vi "ACT_Loop.vi"() -> ()   [LabVIEW 2023, in "RingPlacer_ACT.lvlib"]
uses:
  RingPlacer_ACT.lvlib
  Cluster_CMD_ACT_Data.ctl
  ENUM_Shooter_Mode.ctl
  Cluster_Shooter Status.ctl
  Shooter/Cluster_Speed Sensor Values.ctl
  Shooter/Cluster_Velocity Values.ctl
  Shooter/Cluster_Voltage Values.ctl
  ENUM_ACT_State.ctl
  <vilib>/Rock Robotics/WPI/MotorControl/WPI_MotorControlDeviceRef.ctl
  <vilib>/Rock Robotics/WPI/MotorControl/WPI_MotorControlType.ctl
  <vilib>/Rock Robotics/SystemInterfaces/DIO/FPGA_DIOPWMChannel.ctl
  <vilib>/Rock Robotics/WPI/PWM/WPI_PWMDeadband.ctl
  <vilib>/Rock Robotics/SystemInterfaces/DIO/FPGA_DIOChannel.ctl
  <vilib>/Rock Robotics/WPI/ThirdParty/REV Robotics/REVLib/Typedef/Spark MAX Control Type.ctl
  ENUM_ACT_Action.ctl
  <vilib>/Rock Robotics/WPI/ThirdParty/REV Robotics/REVLib/Typedef/Spark MAX Idle Mode.ctl
  RoboRIO Utilities/Global_STOP.vi
  Global_CMD_ACT_Data In.vi
  Global_ACT_Data Out.vi
  Shooter/Shooter_ACT.lvlib
panel:
  out "Motor Status":T1
  out "Target RPM":dbl
  out "Input DBL Data":T5
  out "Output DBL Data":dbl
  out "Cycle Time (S)":dbl format="%.3g"
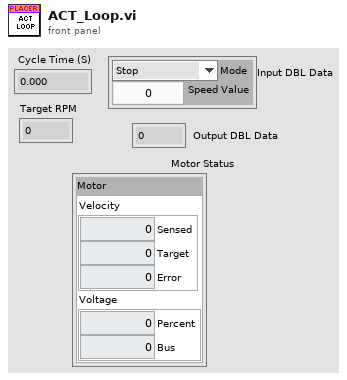
[diagram p1: front panel]
types:
  T1 = typedef "RingPlacer_ACT.lvlib/Cluster_Shooter Status.ctl" = cluster{"Motor":T2}
  T2 = typedef "Cluster_Speed Sensor Values.ctl" = cluster{"Velocity":T3, "Voltage":T4}
  T3 = typedef "Shooter_ACT.lvlib/Cluster_Velocity Values.ctl" = cluster{"Sensed":dbl, "Target":dbl, "Error":dbl}
  T4 = typedef "Shooter_ACT.lvlib/Cluster_Voltage Values.ctl" = cluster{"Percent":dbl, "Bus":dbl}
  T5 = typedef "RingPlacer_ACT.lvlib/Cluster_CMD_ACT_Data.ctl" = cluster{"Mode":T6, "Speed Value":dbl}
  T6 = typedef "RingPlacer_ACT.lvlib/ENUM_Shooter_Mode.ctl" = enum16{"Stop", "Speed Percent", "Speed RPM"}
  T7 = typedef "Spark MAX Control Type.ctl" = enum16{"Percent VBus", "Voltage", "Velocity", "Position", "Smart Motion", "Current", "Smart Velocity"}
  T8 = typedef "WPI_MotorControlDeviceRef.ctl" = cluster{"DeviceStatus":errorcluster, "Type":T9, "PWM":cluster{"PWM Channel":T10, "DeadBand":T11}, "CAN":cluster{"Device Number":u8, "SetOutput VI Ref":variant, "GetOutput VI Ref":variant, "Enable VI Ref":variant, "Disable VI Ref":variant, "Data":variant}, "Invert":bool, "DIO PWM":cluster{"PWM \"Enable\" Channel":T10, "DIOChannel":T12, "PWM Rate":dbl}}
  T9 = typedef "WPI_MotorControlType.ctl" = enum16{"PWM", "CAN", "DIO PWM"}
  T10 = typedef "FPGA_DIOPWMChannel.ctl" = enum8{"PWM 0", "PWM 1", "PWM 2", "PWM 3", "PWM 4", "PWM 5", "PWM 6", "PWM 7", "PWM 8", "PWM 9", "PWM MXP 0", "PWM MXP 1", "PWM MXP 2", "PWM MXP 3", "PWM MXP 4", "PWM MXP 5", "PWM MXP 6", "PWM MXP 7", "PWM MXP 8", "PWM MXP 9", "Invalid"}
  T11 = typedef "WPI_PWMDeadband.ctl" = cluster{"Name":string, "maxPositivePwm":i32, "minPositivePwm":i32, "centerPwm":i32, "maxNegativePwm":i32, "minNegativePwm":i32, "angularRange":u16}
  T12 = typedef "FPGA_DIOChannel.ctl" = enum8{"DIO 0", "DIO 1", "DIO 2", "DIO 3", "DIO 4", "DIO 5", "DIO 6", "DIO 7", "DIO 8", "DIO 9", "DIO MXP 0", "DIO MXP 1", "DIO MXP 2", "DIO MXP 3", "DIO MXP 4", "DIO MXP 5", "DIO MXP 6", "DIO MXP 7", "DIO MXP 8", "DIO MXP 9", "DIO MXP 10", "DIO MXP 11", "DIO MXP 12", "DIO MXP 13", "DIO MXP 14", "DIO MXP 15", "SPI Port CS1", "SPI Port CS2", "SPI Port CS3", "SPI Port MISO", "SPI Port MOSI", "Invalid"}
  T13 = typedef "RingPlacer_ACT.lvlib/ENUM_ACT_State.ctl" = enum16{"Starting", "Stopping", "Shooting", "Shutdown"}
  T14 = typedef "RingPlacer_ACT.lvlib/ENUM_ACT_Action.ctl" = enum16{"No Action", "Reset Time", "Reset All", "Setup Motors", "Setup Sensors", "Stop", "Set Speed RPM", "Set Speed Percent"}
  T15 = cluster{"Motor Ref":T8, "State":T13, "Previous State":T13, "Current Time":timestamp, "Previous Time":timestamp, "Start Time":timestamp, "Target Time (ms)":u32, "Cycle Time(S)":dbl, "ACT Input":T5, "Motor Value":dbl, "Control Mode":T7, "Target RPM":dbl, "Motor Status":T1}
  T16 = typedef "Spark MAX Idle Mode.ctl" = enum16{"Coast", "Brake"}
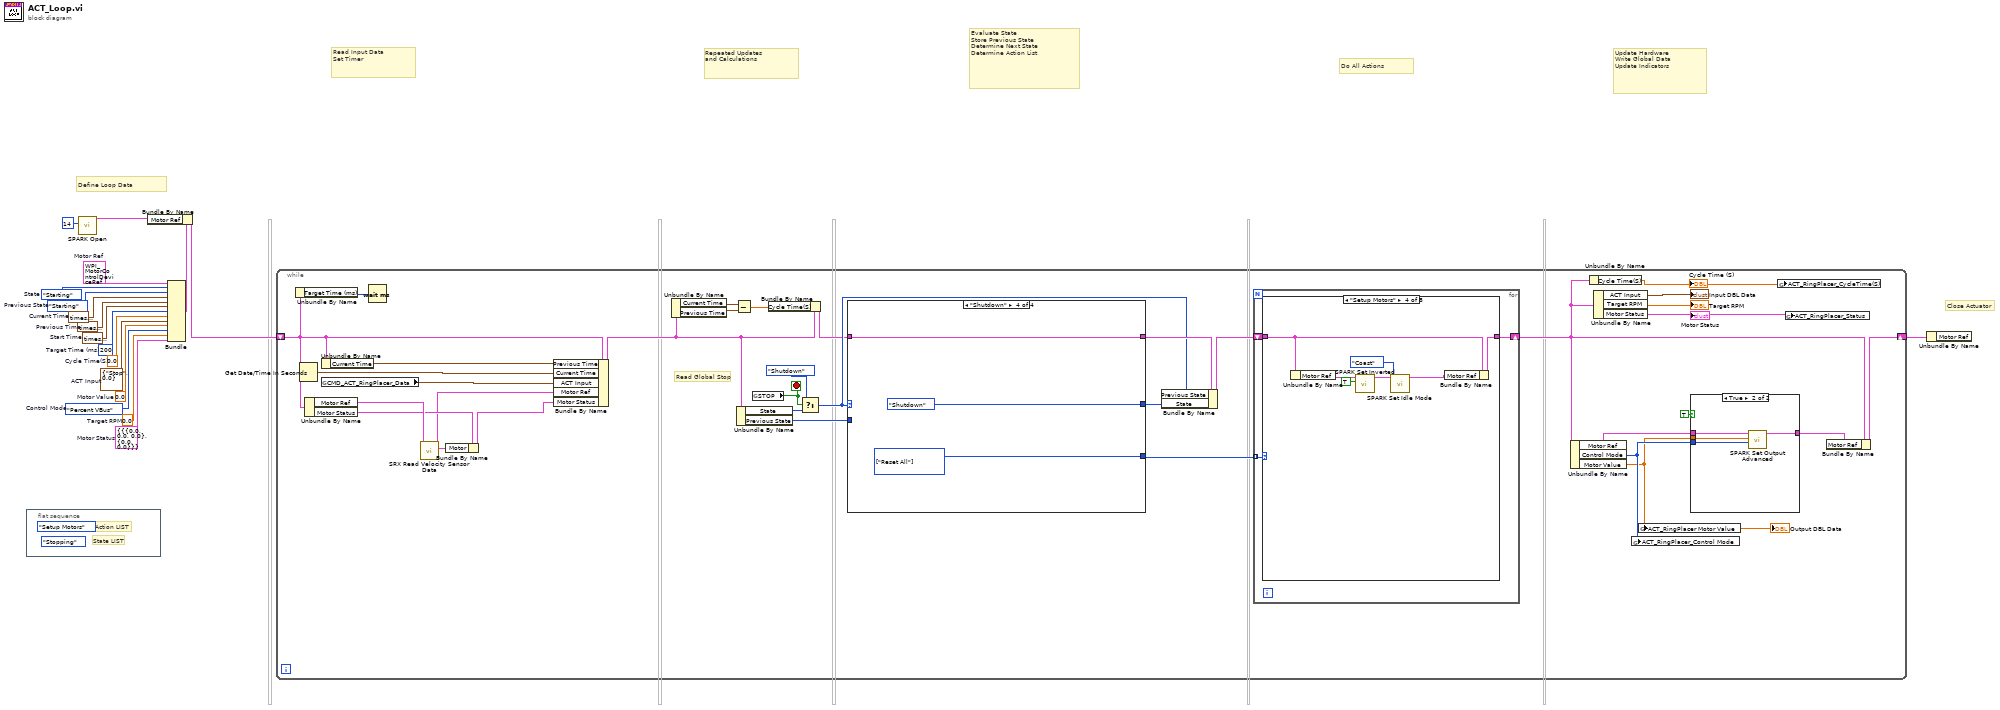
[diagram p0: block diagram]
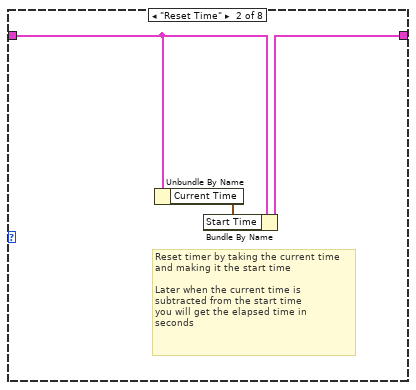
[diagram p4: hidden frame]
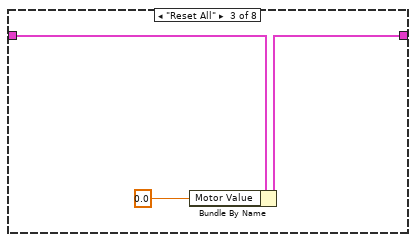
[diagram p5: hidden frame]
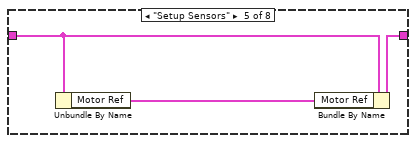
[diagram p6: hidden frame]
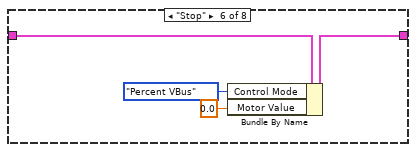
[diagram p7: hidden frame]
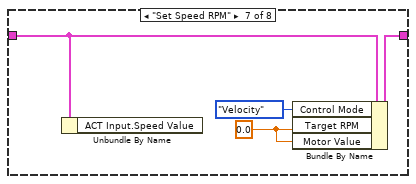
[diagram p8: hidden frame]
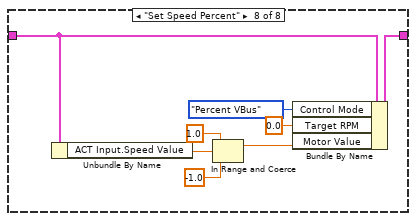
[diagram p9: hidden frame]
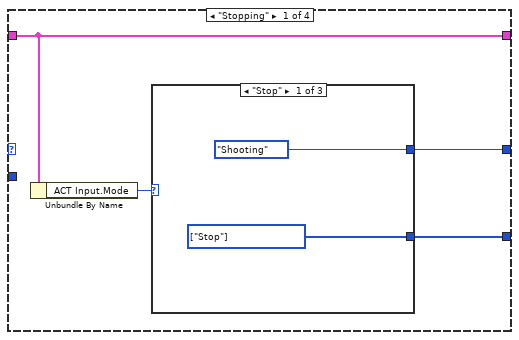
[diagram p10: hidden frame]
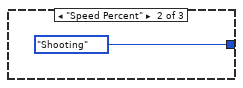
[diagram p11: hidden frame]
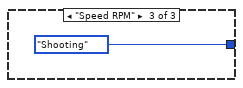
[diagram p12: hidden frame]
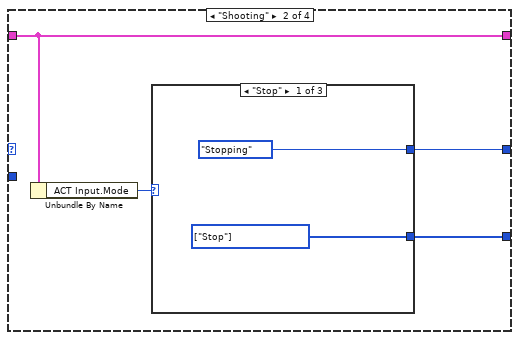
[diagram p13: hidden frame]
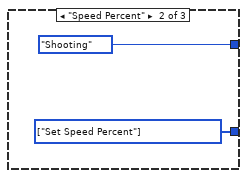
[diagram p14: hidden frame]
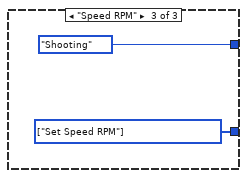
[diagram p15: hidden frame]
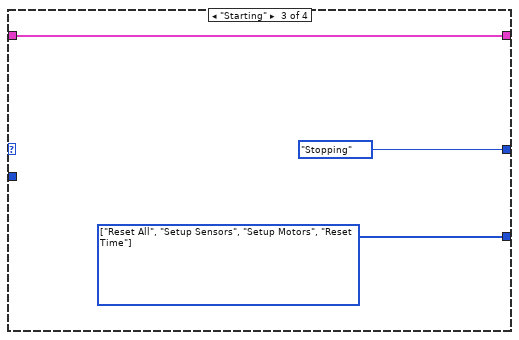
[diagram p16: hidden frame]
diagram:
  w1 = Spark_MAX_Control_Type."Percent VBus"  # Control Mode
  w4 = T1 {"Motor"={"Velocity"={"Sensed"=0.0, "Target"=0.0, "Error"=0.0}, "Voltage"={"Percent"=0.0, "Bus"=0.0}}}  # Motor Status
  w5 = 0.0  # Target RPM
  w6 = T8 {"DeviceStatus"={"status"=FALSE, "code"=0, "source"=""}, "Type"=enum."PWM", "PWM"={"PWM Channel"=enum."PWM 1", "DeadBand"={"Name"="", "maxPositivePwm"=0, "minPositivePwm"=0, "centerPwm"=0, "maxNegativePwm"=0, "minNegativePwm"=0, "angularRange"=0}}, "CAN"={"Device Number"=0, "SetOutput VI Ref"=variant(enum8{"Percent VBus", "Current", "Speed", "Position", "Voltage"} enum."Percent VBus"), "GetOutput VI Ref"=variant(refnum<k1> refnum), "Enable VI Ref"=variant(dbl 12.0), "Disable VI Ref"=variant(enum8{"Percent VBus", "Speed", "Position", "Slave", "Unchanged / Invalid", "Voltage Compensation", "Current", "Motion Profile"} enum."Percent VBus"), "Data"=variant}, "Invert"=FALSE, "DIO PWM"={"PWM \"Enable\" Channel"=enum."Invalid", "DIOChannel"=enum."Invalid", "PWM Rate"=0.0}}  # Motor Ref
  w10 = 0.0  # Cycle Time(S)
  w11 = ENUM_ACT_State."Starting"  # Previous State
  w12 = timestamp(0 s since 1904-01-01)  # Previous Time
  w13 = u32 200  # Target Time (ms)
  w14 = 0.0  # Motor Value
  w15 = T5 {"Mode"=enum."Stop", "Speed Value"=0.0}  # ACT Input
  w16 = timestamp(0 s since 1904-01-01)  # Start Time
  w17 = timestamp(0 s since 1904-01-01)  # Current Time
  w18 = ENUM_ACT_State."Starting"  # State
  # "Close Actuator"
  # "Define Loop Data"
  # "Repeated Updates\nand Calculations"
  # "Read Input Data\nSet Timer"
  # "Evaluate State\nStore Previous State\nDetermine Next State\nDetermine Action List"
  # "Do All Actions"
  # "Update Hardware\nWrite Global Data\nUpdate Indicators"
  n1 = flat-sequence {
    frame #0 {
      (unwired) ENUM_ACT_State."Stopping" ("State")
      (unwired) ENUM_ACT_Action."Setup Motors" ("Action")
      # "State LIST"
      # "Action LIST"
    }
  }
  n2 = call <vilib>:"SPARK Open.vi"("Device Number"=u8 14) -> ("MotorControlDeviceRef"=w3:T8)  [unwired: 9 in, 1 out]
  n3 = Bundle("Motor Ref"=w6, "State"=w18, "Previous State"=w11, "Current Time"=w17, "Previous Time"=w12, "Start Time"=w16, "Target Time (ms)"=w13, "Cycle Time(S)"=w10, "ACT Input"=w15, "Motor Value"=w14, "Control Mode"=w1, "Target RPM"=w5, "Motor Status"=w4) -> (w8:T15)  [unwired: 1 in]
  n4 = Bundle By Name(cluster=w8, "Motor Ref"=w3) -> (w7:T15)
  n5 = while {
    shift-right: [w33] -> w9
    shift-left: w7 -> [w26]
    stop <- w49 stop-if-true
    # "Read Global Stop"
    n6 = Unbundle By Name(w26) -> ("Target Time (ms)"=w46:u32)
    n7 = Get Date/Time In Seconds() -> (seconds since 1Jan1904=w53:timestamp)
    n8 = Unbundle By Name(w26) -> ("Motor Ref"=w25:T8, "Motor Status"=w24:T1)
    n9 = Unbundle By Name(w26) -> ("Current Time"=w45:timestamp)
    n10 = global read "Global_CMD_ACT_Data In.vi" "CMD_ACT_RingPlacer_Data"() -> (w35:T5)
    n11 = Wait (ms)(milliseconds to wait=w46) -> ()  [unwired: 1 out]
    n12 = call "SRX Read Velocity Sensor Data.vi"("SRX Ref"=w25) -> ("Sensor Status Out"=w19:T2, "SRX Ref Out"=w22:T8)  [unwired: 8 in, 1 out]
    n13 = Bundle By Name(cluster=w24, "Motor"=w19) -> (w23:T1)
    n14 = Bundle By Name(cluster=w26, "Previous Time"=w45, "Current Time"=w53, "ACT Input"=w35, "Motor Ref"=w22, "Motor Status"=w23) -> (w40:T15)
    n15 = Unbundle By Name(w40) -> ("Current Time"=w41:timestamp, "Previous Time"=w42:timestamp)
    n16 = Subtract(x=w41, y=w42) -> (x-y=w38:dbl)
    n17 = Unbundle By Name(w40) -> ("State"=w47:T13, "Previous State"=w44:T13)
    n18 = global read "Global_STOP.vi" "STOP"() -> (w49:bool)
    n19 = Bundle By Name(cluster=w40, "Cycle Time(S)"=w38) -> (w39:T15)
    n20 = Select(t=ENUM_ACT_State."Shutdown" ("State"), s=w49, f=w47) -> (s? t:f=w43:T13)
    n21 = case shown="\"Shutdown\"" w43 {
      tunnel: w39 -> [w96 w104 w115 w118]
      tunnel: [w96 w104 w115 w118] -> w51
      tunnel: [w97 w105 ENUM_ACT_State."Stopping" ("State") ENUM_ACT_State."Shutdown" ("State")] -> w50
      tunnel: [w98 w106 w113 w116] -> w37
      tunnel: w44 -> [_ _ _ _]
      frame "Stopping" {
        n22 = Unbundle By Name(w96) -> ("ACT Input.Mode"=w95:T6)
        n23 = case shown="\"Stop\"" w95 {
          tunnel: [w100 _ _] -> w98
          tunnel: [ENUM_ACT_State."Shooting" ("State") ENUM_ACT_State."Shooting" ("State") ENUM_ACT_State."Shooting" ("State")] -> w97
          frame "Stop" {
            w100 = T14[] [enum."Stop"] items=["No Action", "Reset Time", "Reset All", "Setup Motors", "Setup Sensors", "Stop", "Set Speed RPM", "Set Speed Percent"] ("Actions")
          }
          frame "Speed Percent" {
          }
          frame "Speed RPM" {
          }
        }
      }
      frame "Shooting" {
        n24 = Unbundle By Name(w104) -> ("ACT Input.Mode"=w103:T6)
        n25 = case shown="\"Stop\"" w103 {
          tunnel: [w107 w109 w111] -> w106
          tunnel: [ENUM_ACT_State."Stopping" ("State") ENUM_ACT_State."Shooting" ("State") ENUM_ACT_State."Shooting" ("State")] -> w105
          frame "Stop" {
            w107 = T14[] [enum."Stop"] items=["No Action", "Reset Time", "Reset All", "Setup Motors", "Setup Sensors", "Stop", "Set Speed RPM", "Set Speed Percent"] ("Actions")
          }
          frame "Speed Percent" {
            w109 = T14[] [enum."Set Speed Percent"] items=["No Action", "Reset Time", "Reset All", "Setup Motors", "Setup Sensors", "Stop", "Set Speed RPM", "Set Speed Percent"] ("Actions")
          }
          frame "Speed RPM" {
            w111 = T14[] [enum."Set Speed RPM"] items=["No Action", "Reset Time", "Reset All", "Setup Motors", "Setup Sensors", "Stop", "Set Speed RPM", "Set Speed Percent"] ("Actions")
          }
        }
      }
      frame "Starting" {
        w113 = T14[] [enum."Reset All", enum."Setup Sensors", enum."Setup Motors", enum."Reset Time"] items=["No Action", "Reset Time", "Reset All", "Setup Motors", "Setup Sensors", "Stop", "Set Speed RPM", "Set Speed Percent"] ("Actions")
      }
      frame "Shutdown" {
        w116 = T14[] [enum."Reset All"] items=["No Action", "Reset Time", "Reset All", "Setup Motors", "Setup Sensors", "Stop", "Set Speed RPM", "Set Speed Percent"] ("Actions")
      }
    }
    n26 = Bundle By Name(cluster=w51, "Previous State"=w43, "State"=w50) -> (w52:T15)
    n27 = for {
      tunnel: w37 -> [w61] mode=indexing
      shift-right: [w60] -> w34
      shift-left: w52 -> [w59]
      n28 = case shown="\"Setup Motors\"" w61 {
        tunnel: w59 -> [w62 w65 w68 w75 w78 w81 w85 w93]
        tunnel: [w62 w64 w67 w74 w77 w82 w86 w94] -> w60
        frame "No Action" {
        }
        frame "Reset Time" {
          # "Reset timer by taking the current time\nand making it the start time\n\nLater when the current time is \nsubtracted from the start time\nyou will get the elapsed time in \nseconds"
          n29 = Unbundle By Name(w65) -> ("Current Time"=w63:timestamp)
          n30 = Bundle By Name(cluster=w65, "Start Time"=w63) -> (w64:T15)
        }
        frame "Reset All" {
          n31 = Bundle By Name(cluster=w68, "Motor Value"=0.0 ("FG Write Value")) -> (w67:T15)
        }
        frame "Setup Motors" {
          n32 = Unbundle By Name(w75) -> ("Motor Ref"=w73:T8)
          n33 = call <vilib>:"SPARK Set Inverted.vi"("Inverted (F)"=TRUE, "MotorControlDeviceRef in"=w73) -> ("MotorControlDeviceRef out"=w71:T8)  [unwired: 8 in, 1 out]
          n34 = call <vilib>:"SPARK Set Idle Mode.vi"("Idle Mode"=Spark_MAX_Idle_Mode."Coast", "MotorControlDeviceRef in"=w71) -> ("MotorControlDeviceRef out"=w70:T8)  [unwired: 8 in, 1 out]
          n35 = Bundle By Name(cluster=w75, "Motor Ref"=w70) -> (w74:T15)
        }
        frame "Setup Sensors" {
          n36 = Unbundle By Name(w78) -> ("Motor Ref"=w76:T8)
          n37 = Bundle By Name(cluster=w78, "Motor Ref"=w76) -> (w77:T15)
        }
        frame "Stop" {
          n38 = Bundle By Name(cluster=w81, "Control Mode"=Spark_MAX_Control_Type."Percent VBus", "Motor Value"=0.0) -> (w82:T15)
        }
        frame "Set Speed RPM" {
          w84 = 0.0 ("Target RPM")
          n39 = Unbundle By Name(w85) -> ()  [unwired: 1 out]
          n40 = Bundle By Name(cluster=w85, "Control Mode"=Spark_MAX_Control_Type."Velocity", "Target RPM"=w84, "Motor Value"=w84) -> (w86:T15)
        }
        frame "Set Speed Percent" {
          n41 = Unbundle By Name(w93) -> ("ACT Input.Speed Value"=w91:dbl)
          n42 = In Range and Coerce(upper limit=1.0, x=w91, lower limit=-1.0 ("upper limit")) -> (coerced(x)=w88:dbl)  [unwired: 1 out]
          n43 = Bundle By Name(cluster=w93, "Control Mode"=Spark_MAX_Control_Type."Percent VBus", "Target RPM"=0.0, "Motor Value"=w88) -> (w94:T15)
        }
      }
    }
    n44 = Unbundle By Name(w34) -> ("Motor Ref"=w31:T8, "Control Mode"=w29:T7, "Motor Value"=w28:dbl)
    "Output DBL Data" <- w28
    n45 = Unbundle By Name(w34) -> ("Cycle Time(S)"=w32:dbl)
    "Cycle Time (S)" <- w32
    n46 = Unbundle By Name(w34) -> ("ACT Input"=→"Input DBL Data":T5, "Target RPM"=→"Target RPM":dbl, "Motor Status"=w21:T1)
    "Motor Status" <- w21
    n47 = global write "Global_ACT_Data Out.vi" "ACT_RingPlacer_Control Mode"(w29) -> ()
    n48 = global write "Global_ACT_Data Out.vi" "ACT_RingPlacer Motor Value"(w28) -> ()
    n49 = case shown="True" TRUE {
      tunnel: w31 -> [w54 w58]
      tunnel: [w54 w57] -> w30
      tunnel: w29 -> [_ w56]
      tunnel: w28 -> [_ w55]
      frame False {
      }
      frame True {
        n50 = call <vilib>:"SPARK Set Output Advanced.vi"("Control Mode"=w56, "Setpoint"=w55, "MotorControlDevRef"=w58) -> ("MotorControlDevRef"=w57:T8)  [unwired: 7 in, 1 out]
      }
    }
    n51 = global write "Global_ACT_Data Out.vi" "ACT_RingPlacer_CycleTime(S)"(w32) -> ()
    n52 = global write "Global_ACT_Data Out.vi" "ACT_RingPlacer_Status"(w21) -> ()
    n53 = Bundle By Name(cluster=w34, "Motor Ref"=w30) -> (w33:T15)
  }
  n54 = Unbundle By Name(w9) -> ()  [unwired: 1 out]
